vi "Test Geometry Location Fitting.vi"() -> ()   [LabVIEW 2011]
uses:
  <vilib>/Analysis/Matrix/Datatypes/RealMatrix.ctl
  Orient3d Class/Type Definitions/Quaternion.ctl
  Type Definitions/Position_Orientation.ctl
  Vec3d Class/Vec3d Class.lvclass
  Orient3d Class/Orient3d Class.lvclass
  <vilib>/gmath/statdist.llb/Normal Random.vi
  <vilib>/gmath/NI_Gmath.lvlib
  <vilib>/Analysis/Matrix/NI_Matrix.lvlib
panel:
  in  "Quaternion In":T1={"x"=0.0, "y"=0.0, "z"=1.0, "w"=1.0}
  out "Quaternion Result":T1
  in  "Scale-Z\n(mm)":dbl=1.0
  out "Rotation Matrix Out":T2 format="%.4f"
  out "Rotation Matrix In":T2 format="%.4f"
  out "error out":errorcluster
  out "residual":dbl format="%_4e"
  out "offset":cluster{"x":dbl, "y":dbl, "z":dbl} {"x" format="%_4e"; "y" format="%_4e"; "z" format="%_4e"}
  in  "Scale\n(mm)":dbl=100.0
  in  "Offset\n(mm)":cluster{"x":dbl, "y":dbl, "z":dbl}
  in  "Noise\n(mm)":dbl=10.0
  in  "Sample Size":u32=1000
  # "Fitted Values"
  # "Input Values"
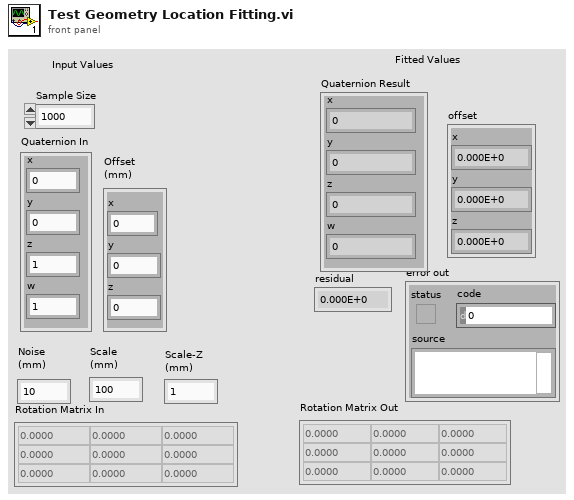
[diagram p1: front panel]
types:
  T1 = typedef "Quaternion.ctl" = cluster{"x":dbl, "y":dbl, "z":dbl, "w":dbl}
  T2 = typedef "NI_Matrix.lvlib/RealMatrix.ctl" = dbl[][]
  T3 = typedef "Position_Orientation.ctl" = cluster{"Center":refnum<class "Vec3d Class.lvclass">, "Orientation":refnum<class "Orient3d Class.lvclass">}
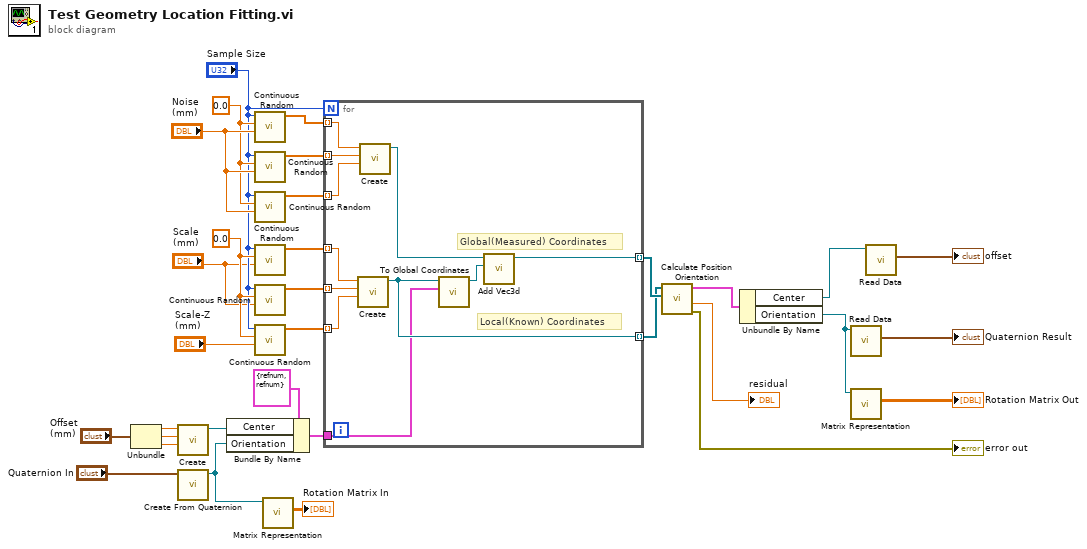
[diagram p0: block diagram]
diagram:
  w27 = 0.0 ("mean")
  w30 = 0.0 ("mean")
  n1 = Unbundle("Offset\n(mm)") -> ("x"=w18:dbl, "y"=w19:dbl, "z"=w20:dbl)
  n2 = call "Create.vi"("Z"=w20, "Y"=w19, "X"=w18) -> ("Vec3d Class out"=w16:refnum<class "Vec3d Class.lvclass">)  [unwired: 7 in, 1 out]
  n3 = call "Create From Quaternion.vi"("Quaternion"="Quaternion In") -> ("Orient3d out"=w2:refnum<class "Orient3d Class.lvclass">)  [unwired: 9 in, 1 out]
  n4 = Bundle By Name(cluster=T3 {"Center"=refnum, "Orientation"=refnum} ("Center/Orientation"), "Center"=w16, "Orientation"=w2) -> (w15:T3)
  n5 = call-poly <vilib>:"Continuous Random.vi"("std"="Noise\n(mm)", "mean"=w30, "samples"="Sample Size") -> ("normal random data"=w32:dbl[])  [unwired: 7 in, 1 out]
  n6 = call-poly <vilib>:"Continuous Random.vi"("std"="Noise\n(mm)", "mean"=w30, "samples"="Sample Size") -> ("normal random data"=w29:dbl[])  [unwired: 7 in, 1 out]
  n7 = call-poly <vilib>:"Continuous Random.vi"("std"="Noise\n(mm)", "mean"=w30, "samples"="Sample Size") -> ("normal random data"=w28:dbl[])  [unwired: 7 in, 1 out]
  n8 = call-poly <vilib>:"Continuous Random.vi"("std"="Scale\n(mm)", "mean"=w27, "samples"="Sample Size") -> ("normal random data"=w24:dbl[])  [unwired: 7 in, 1 out]
  n9 = call-poly <vilib>:"Continuous Random.vi"("std"="Scale\n(mm)", "mean"=w27, "samples"="Sample Size") -> ("normal random data"=w23:dbl[])  [unwired: 7 in, 1 out]
  n10 = call-poly <vilib>:"Continuous Random.vi"("std"="Scale-Z\n(mm)", "mean"=w27, "samples"="Sample Size") -> ("normal random data"=w22:dbl[])  [unwired: 7 in, 1 out]
  n11 = call "Matrix Representation.vi"("Orient3d in"=w2) -> ("Rotation Matrix"=→"Rotation Matrix In":T2)  [unwired: 8 in, 2 out]
  n12 = for {
    N: "Sample Size" -> [_]
    tunnel: w32 -> [w43] mode=indexing
    tunnel: w29 -> [w42] mode=indexing
    tunnel: w28 -> [w41] mode=indexing
    tunnel: w24 -> [w40] mode=indexing
    tunnel: w23 -> [w39] mode=indexing
    tunnel: w22 -> [w38] mode=indexing
    tunnel: w15 -> [w33]
    tunnel: [w36] -> w6 mode=indexing
    tunnel: [w34] -> w5 mode=indexing
    # "Global(Measured) Coordinates"
    # "Local(Known) Coordinates"
    n13 = call "Create.vi"("Z"=w38, "Y"=w39, "X"=w40) -> ("Vec3d Class out"=w34:refnum<class "Vec3d Class.lvclass">)  [unwired: 7 in, 1 out]
    n14 = call "Create.vi"("Z"=w41, "Y"=w42, "X"=w43) -> ("Vec3d Class out"=w37:refnum<class "Vec3d Class.lvclass">)  [unwired: 7 in, 1 out]
    n15 = call "To Global Coordinates.vi"("Center/Orientation"=w33, "Local Coordinates"=w34) -> ("Global Coordinates"=w35:refnum<class "Vec3d Class.lvclass">)  [unwired: 8 in, 1 out]
    n16 = call-dynamic "Add Vec3d.vi"(10:"Vec3d Class in"=w35, 11:"Vec3d Class in"=w37) -> ("Vec3d Class out"=w36:refnum<class "Vec3d Class.lvclass">)  [unwired: 8 in, 1 out]
  }
  n17 = call "Calculate Position Orientation.vi"("Measured Global Positions"=w6, "Known Local Positions"=w5) -> ("error out"=→"error out":errorcluster, "Residual"=→"residual":dbl, "PositionOrientation"=w8:T3)  [unwired: 7 in]
  n18 = Unbundle By Name(w8) -> ("Center"=w13:refnum<class "Vec3d Class.lvclass">, "Orientation"=w10:refnum<class "Orient3d Class.lvclass">)
  n19 = call "Read Data.vi"("Orient3d in"=w10) -> ("Quaternion"=→"Quaternion Result":T1)  [unwired: 8 in, 2 out]
  n20 = call "Matrix Representation.vi"("Orient3d in"=w10) -> ("Rotation Matrix"=→"Rotation Matrix Out":T2)  [unwired: 8 in, 2 out]
  n21 = call-dynamic "Read Data.vi"("Vec3d Class in"=w13) -> ("Data"=→"offset":cluster{"X":dbl, "Y":dbl, "Z":dbl})  [unwired: 8 in, 2 out]
